vi "Guarda_Datos.vi"(0 "Texto (I)":string, 1 "Ruta":path, 2 "Operación":T1(ring), 3 "Acceso":enum16{"read/write", "read-only", "write-only"}(ring), 4 "Error (I)":errorcluster) -> (5 "Texto (O)":string, 6 "Error (O)":errorcluster)   [LabVIEW 2020]
doc: "Selecciona la operación que se quiere ejecutar sobre el archivo especificado en la ruta y el tipo de acceso que se desea tener a él, para escribir el texto entregado y/o leer el texto en el mismo. La operación de lectura y escritura ocurre en ese orden: lectura y luego escritura.\n\nTexto (I): Texto que será escrito al final del archivo.\n\nRuta: Ruta del archivo (el archivo mismo y su extensión es parte de la ruta).\n\nOperación: 0 - Abrir; 1 - Reemplazar; 2 - Crear; 3 - Abrir o crear; 4 - Reemplazar o crear; 5 - Reemplazar o creear con confirmación.\n\nAcceso: 0 - Leer y Escribir; 1 - Leer; 2 - Escribir.\n\nError (I): Ingreso de errores previos.\n\nTexto (O): Texto contenido en el archivo antes de escribirle el nuevo texto en Texto (I). Devuelve un string explicando un error en caso de que el Acceso no permita la opción de Leer.\n\nError (O): Salida de errores previos más los de esta VI."
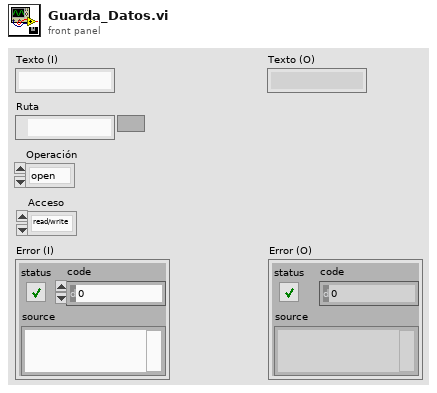
[diagram p1: front panel]
types:
  T1 = enum16{"open", "replace", "create", "open or create", "replace or create", "replace or create with confirmation"}
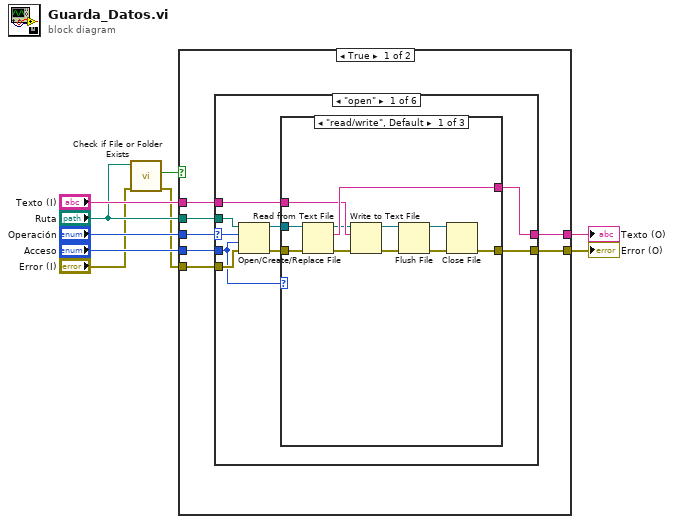
[diagram p0: block diagram]
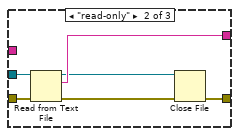
[diagram p2: hidden frame]
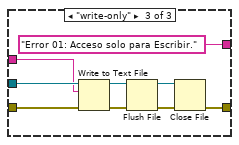
[diagram p3: hidden frame]
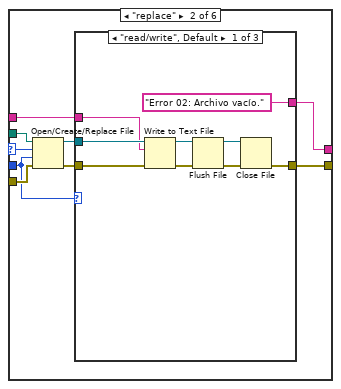
[diagram p4: hidden frame]
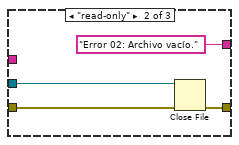
[diagram p5: hidden frame]
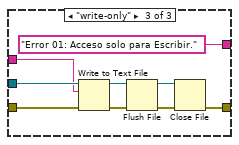
[diagram p6: hidden frame]
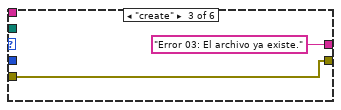
[diagram p7: hidden frame]
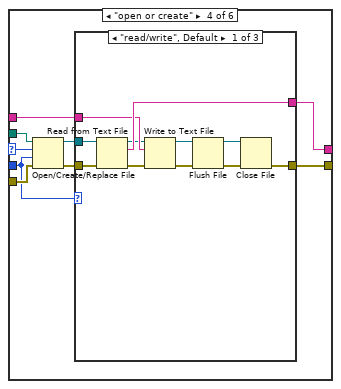
[diagram p8: hidden frame]
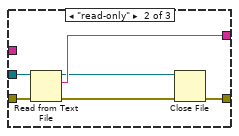
[diagram p9: hidden frame]
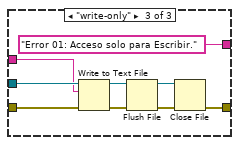
[diagram p10: hidden frame]
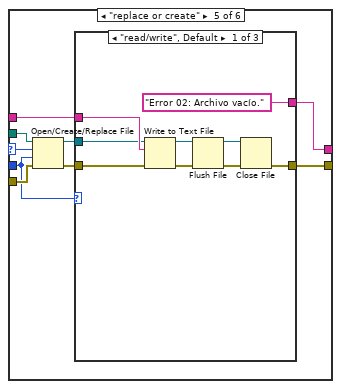
[diagram p11: hidden frame]
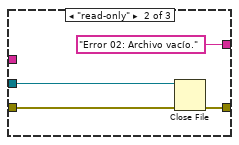
[diagram p12: hidden frame]
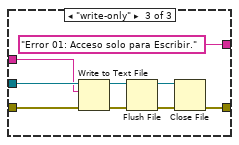
[diagram p13: hidden frame]
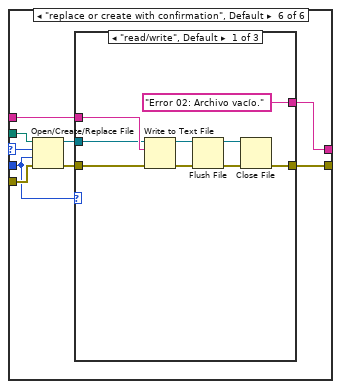
[diagram p14: hidden frame]
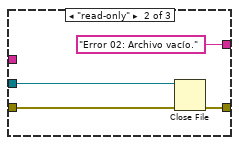
[diagram p15: hidden frame]
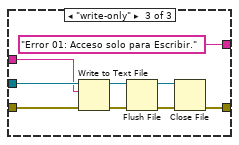
[diagram p16: hidden frame]
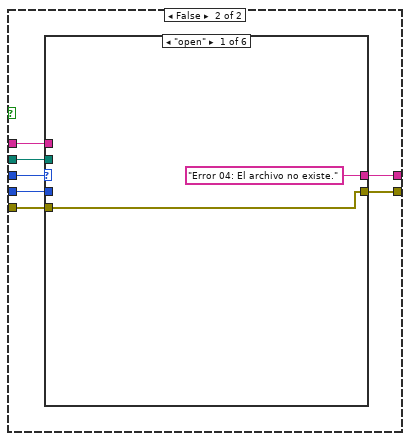
[diagram p17: hidden frame]
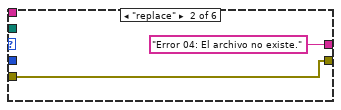
[diagram p18: hidden frame]
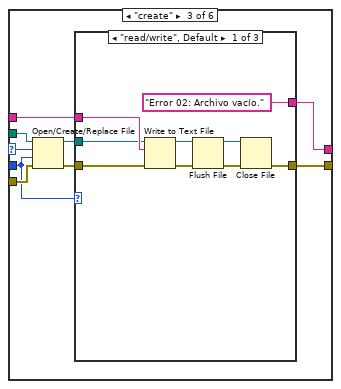
[diagram p19: hidden frame]
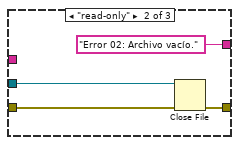
[diagram p20: hidden frame]
diagram:
  n1 = call <vilib>:"Check if File or Folder Exists.vi"("error in (no error)"="Error (I)", "path"="Ruta") -> ("error out"=w1:errorcluster, "file or folder exists?"=w3:bool)  [unwired: 7 in, 1 out]
  n2 = case shown="True" w3 {
    tunnel: "Operación" -> [w16 w188]
    tunnel: "Ruta" -> [w15 w187]
    tunnel: "Acceso" -> [w14 w186]
    tunnel: w1 -> [w13 w185]
    tunnel: "Texto (I)" -> [w12 w184]
    tunnel: [w11 w183] -> w6
    tunnel: [w10 w182] -> w5
    frame True {
      n3 = case shown="\"open\"" w16 {
        selector: w16 -> [w25 w60 _ w93 w128 w159]
        tunnel: w15 -> [w24 w59 _ w92 w127 w158]
        tunnel: w14 -> [w22 w57 _ w90 w125 w156]
        tunnel: w13 -> [w23 w58 w84 w91 w126 w157]
        tunnel: w12 -> [w19 w54 _ w87 w122 w153]
        tunnel: [w18 w53 w84 w86 w121 w152] -> w11
        tunnel: [w17 w52 "Error 03: El archivo ya existe." ("Texto (I)") w85 w120 w151] -> w10
        frame "open" {
          n4 = Open/Create/Replace File(file path (use dialog)=w24, error in=w23, operation (0:open)=w25, access (0:read/write)=w22) -> (refnum out=w21:refnum<file>, error out=w20:errorcluster)  [unwired: 2 in, 1 out]
          n5 = case shown="\"read/write\", Default" w22 {
            tunnel: w21 -> [w36 w42 w46]
            tunnel: w20 -> [w35 w41 w45]
            tunnel: [w34 w40 "Error 01: Acceso solo para Escribir."] -> w17
            tunnel: w19 -> [w33 _ w44]
            tunnel: [w26 w39 w47] -> w18
            frame "read/write", Default {
              n6 = Read from Text File(file (use dialog)=w36, error in=w35) -> (refnum out=w32:refnum<file>, text=w34:string, error out=w31:errorcluster)  [unwired: 2 in, 1 out]
              n7 = Write to Text File(file (use dialog)=w32, text=w33, error in=w31) -> (refnum out=w30:refnum<file>, error out=w29:errorcluster)  [unwired: 1 in, 1 out]
              n8 = Flush File(refnum=w30, error in=w29) -> (refnum out=w28:refnum<file>, error out=w27:errorcluster)
              n9 = Close File(refnum=w28, error in=w27) -> (error out=w26:errorcluster)  [unwired: 1 out]
            }
            frame "read-only" {
              n10 = Read from Text File(file (use dialog)=w42, error in=w41) -> (refnum out=w37:refnum<file>, text=w40:string, error out=w38:errorcluster)  [unwired: 2 in, 1 out]
              n11 = Close File(refnum=w37, error in=w38) -> (error out=w39:errorcluster)  [unwired: 1 out]
            }
            frame "write-only" {
              n12 = Write to Text File(file (use dialog)=w46, text=w44, error in=w45) -> (refnum out=w51:refnum<file>, error out=w50:errorcluster)  [unwired: 1 in, 1 out]
              n13 = Flush File(refnum=w51, error in=w50) -> (refnum out=w49:refnum<file>, error out=w48:errorcluster)
              n14 = Close File(refnum=w49, error in=w48) -> (error out=w47:errorcluster)  [unwired: 1 out]
            }
          }
        }
        frame "replace" {
          n15 = Open/Create/Replace File(file path (use dialog)=w59, error in=w58, operation (0:open)=w60, access (0:read/write)=w57) -> (refnum out=w56:refnum<file>, error out=w55:errorcluster)  [unwired: 2 in, 1 out]
          n16 = case shown="\"read/write\", Default" w57 {
            tunnel: w56 -> [w65 w71 w77]
            tunnel: w55 -> [w64 w72 w76]
            tunnel: ["Error 02: Archivo vacío." ("Texto (I)") "Error 02: Archivo vacío." ("Texto (I)") "Error 01: Acceso solo para Escribir." ("Texto (I)")] -> w52
            tunnel: w54 -> [w62 _ w75]
            tunnel: [w63 w70 w78] -> w53
            frame "read/write", Default {
              n17 = Write to Text File(file (use dialog)=w65, text=w62, error in=w64) -> (refnum out=w69:refnum<file>, error out=w68:errorcluster)  [unwired: 1 in, 1 out]
              n18 = Flush File(refnum=w69, error in=w68) -> (refnum out=w67:refnum<file>, error out=w66:errorcluster)
              n19 = Close File(refnum=w67, error in=w66) -> (error out=w63:errorcluster)  [unwired: 1 out]
            }
            frame "read-only" {
              n20 = Close File(refnum=w71, error in=w72) -> (error out=w70:errorcluster)  [unwired: 1 out]
            }
            frame "write-only" {
              n21 = Write to Text File(file (use dialog)=w77, text=w75, error in=w76) -> (refnum out=w82:refnum<file>, error out=w81:errorcluster)  [unwired: 1 in, 1 out]
              n22 = Flush File(refnum=w82, error in=w81) -> (refnum out=w80:refnum<file>, error out=w79:errorcluster)
              n23 = Close File(refnum=w80, error in=w79) -> (error out=w78:errorcluster)  [unwired: 1 out]
            }
          }
        }
        frame "create" {
        }
        frame "open or create" {
          n24 = Open/Create/Replace File(file path (use dialog)=w92, error in=w91, operation (0:open)=w93, access (0:read/write)=w90) -> (refnum out=w89:refnum<file>, error out=w88:errorcluster)  [unwired: 2 in, 1 out]
          n25 = case shown="\"read/write\", Default" w90 {
            tunnel: w89 -> [w104 w110 w114]
            tunnel: w88 -> [w103 w109 w113]
            tunnel: [w102 w108 "Error 01: Acceso solo para Escribir."] -> w85
            tunnel: w87 -> [w101 _ w112]
            tunnel: [w94 w107 w115] -> w86
            frame "read/write", Default {
              n26 = Read from Text File(file (use dialog)=w104, error in=w103) -> (refnum out=w100:refnum<file>, text=w102:string, error out=w99:errorcluster)  [unwired: 2 in, 1 out]
              n27 = Write to Text File(file (use dialog)=w100, text=w101, error in=w99) -> (refnum out=w98:refnum<file>, error out=w97:errorcluster)  [unwired: 1 in, 1 out]
              n28 = Flush File(refnum=w98, error in=w97) -> (refnum out=w96:refnum<file>, error out=w95:errorcluster)
              n29 = Close File(refnum=w96, error in=w95) -> (error out=w94:errorcluster)  [unwired: 1 out]
            }
            frame "read-only" {
              n30 = Read from Text File(file (use dialog)=w110, error in=w109) -> (refnum out=w105:refnum<file>, text=w108:string, error out=w106:errorcluster)  [unwired: 2 in, 1 out]
              n31 = Close File(refnum=w105, error in=w106) -> (error out=w107:errorcluster)  [unwired: 1 out]
            }
            frame "write-only" {
              n32 = Write to Text File(file (use dialog)=w114, text=w112, error in=w113) -> (refnum out=w119:refnum<file>, error out=w118:errorcluster)  [unwired: 1 in, 1 out]
              n33 = Flush File(refnum=w119, error in=w118) -> (refnum out=w117:refnum<file>, error out=w116:errorcluster)
              n34 = Close File(refnum=w117, error in=w116) -> (error out=w115:errorcluster)  [unwired: 1 out]
            }
          }
        }
        frame "replace or create" {
          n35 = Open/Create/Replace File(file path (use dialog)=w127, error in=w126, operation (0:open)=w128, access (0:read/write)=w125) -> (refnum out=w124:refnum<file>, error out=w123:errorcluster)  [unwired: 2 in, 1 out]
          n36 = case shown="\"read/write\", Default" w125 {
            tunnel: w124 -> [w131 w138 w145]
            tunnel: w123 -> [w130 w140 w144]
            tunnel: ["Error 02: Archivo vacío." ("Texto (I)") "Error 02: Archivo vacío." ("Texto (I)") "Error 01: Acceso solo para Escribir." ("Texto (I)")] -> w120
            tunnel: w122 -> [w132 _ w143]
            tunnel: [w133 w139 w146] -> w121
            frame "read/write", Default {
              n37 = Write to Text File(file (use dialog)=w131, text=w132, error in=w130) -> (refnum out=w137:refnum<file>, error out=w136:errorcluster)  [unwired: 1 in, 1 out]
              n38 = Flush File(refnum=w137, error in=w136) -> (refnum out=w135:refnum<file>, error out=w134:errorcluster)
              n39 = Close File(refnum=w135, error in=w134) -> (error out=w133:errorcluster)  [unwired: 1 out]
            }
            frame "read-only" {
              n40 = Close File(refnum=w138, error in=w140) -> (error out=w139:errorcluster)  [unwired: 1 out]
            }
            frame "write-only" {
              n41 = Write to Text File(file (use dialog)=w145, text=w143, error in=w144) -> (refnum out=w150:refnum<file>, error out=w149:errorcluster)  [unwired: 1 in, 1 out]
              n42 = Flush File(refnum=w150, error in=w149) -> (refnum out=w148:refnum<file>, error out=w147:errorcluster)
              n43 = Close File(refnum=w148, error in=w147) -> (error out=w146:errorcluster)  [unwired: 1 out]
            }
          }
        }
        frame "replace or create with confirmation", Default {
          n44 = Open/Create/Replace File(file path (use dialog)=w158, error in=w157, operation (0:open)=w159, access (0:read/write)=w156) -> (refnum out=w155:refnum<file>, error out=w154:errorcluster)  [unwired: 2 in, 1 out]
          n45 = case shown="\"read/write\", Default" w156 {
            tunnel: w155 -> [w162 w169 w176]
            tunnel: w154 -> [w161 w170 w175]
            tunnel: ["Error 02: Archivo vacío." ("Texto (I)") "Error 02: Archivo vacío." ("Texto (I)") "Error 01: Acceso solo para Escribir." ("Texto (I)")] -> w151
            tunnel: w153 -> [w163 _ w174]
            tunnel: [w164 w171 w177] -> w152
            frame "read/write", Default {
              n46 = Write to Text File(file (use dialog)=w162, text=w163, error in=w161) -> (refnum out=w168:refnum<file>, error out=w167:errorcluster)  [unwired: 1 in, 1 out]
              n47 = Flush File(refnum=w168, error in=w167) -> (refnum out=w166:refnum<file>, error out=w165:errorcluster)
              n48 = Close File(refnum=w166, error in=w165) -> (error out=w164:errorcluster)  [unwired: 1 out]
            }
            frame "read-only" {
              n49 = Close File(refnum=w169, error in=w170) -> (error out=w171:errorcluster)  [unwired: 1 out]
            }
            frame "write-only" {
              n50 = Write to Text File(file (use dialog)=w176, text=w174, error in=w175) -> (refnum out=w181:refnum<file>, error out=w180:errorcluster)  [unwired: 1 in, 1 out]
              n51 = Flush File(refnum=w181, error in=w180) -> (refnum out=w179:refnum<file>, error out=w178:errorcluster)
              n52 = Close File(refnum=w179, error in=w178) -> (error out=w177:errorcluster)  [unwired: 1 out]
            }
          }
        }
      }
    }
    frame False {
      n53 = case shown="\"open\"" w188 {
        selector: w188 -> [_ _ w200 w232 w263 w294]
        tunnel: w187 -> [_ _ w198 w231 w262 w293]
        tunnel: w186 -> [_ _ w194 w229 w260 w291]
        tunnel: w185 -> [w190 w192 w197 w230 w261 w292]
        tunnel: w184 -> [_ _ w199 w226 w257 w288]
        tunnel: [w190 w192 w201 w225 w256 w287] -> w183
        tunnel: ["Error 04: El archivo no existe." ("Texto (I)") "Error 04: El archivo no existe." ("Texto (I)") w193 w224 w255 w286] -> w182
        frame "open" {
        }
        frame "replace" {
        }
        frame "create" {
          n54 = Open/Create/Replace File(file path (use dialog)=w198, error in=w197, operation (0:open)=w200, access (0:read/write)=w194) -> (refnum out=w196:refnum<file>, error out=w195:errorcluster)  [unwired: 2 in, 1 out]
          n55 = case shown="\"read/write\", Default" w194 {
            tunnel: w196 -> [w203 w212 w218]
            tunnel: w195 -> [w202 w211 w217]
            tunnel: ["Error 02: Archivo vacío." "Error 02: Archivo vacío." "Error 01: Acceso solo para Escribir."] -> w193
            tunnel: w199 -> [w210 _ w216]
            tunnel: [w205 w214 w219] -> w201
            frame "read/write", Default {
              n56 = Write to Text File(file (use dialog)=w203, text=w210, error in=w202) -> (refnum out=w209:refnum<file>, error out=w208:errorcluster)  [unwired: 1 in, 1 out]
              n57 = Flush File(refnum=w209, error in=w208) -> (refnum out=w207:refnum<file>, error out=w206:errorcluster)
              n58 = Close File(refnum=w207, error in=w206) -> (error out=w205:errorcluster)  [unwired: 1 out]
            }
            frame "read-only" {
              n59 = Close File(refnum=w212, error in=w211) -> (error out=w214:errorcluster)  [unwired: 1 out]
            }
            frame "write-only" {
              n60 = Write to Text File(file (use dialog)=w218, text=w216, error in=w217) -> (refnum out=w223:refnum<file>, error out=w222:errorcluster)  [unwired: 1 in, 1 out]
              n61 = Flush File(refnum=w223, error in=w222) -> (refnum out=w221:refnum<file>, error out=w220:errorcluster)
              n62 = Close File(refnum=w221, error in=w220) -> (error out=w219:errorcluster)  [unwired: 1 out]
            }
          }
        }
        frame "open or create" {
          n63 = Open/Create/Replace File(file path (use dialog)=w231, error in=w230, operation (0:open)=w232, access (0:read/write)=w229) -> (refnum out=w228:refnum<file>, error out=w227:errorcluster)  [unwired: 2 in, 1 out]
          n64 = case shown="\"read/write\", Default" w229 {
            tunnel: w228 -> [w235 w244 w249]
            tunnel: w227 -> [w234 w243 w248]
            tunnel: ["Error 02: Archivo vacío." "Error 02: Archivo vacío." "Error 01: Acceso solo para Escribir."] -> w224
            tunnel: w226 -> [w241 _ w247]
            tunnel: [w236 w245 w250] -> w225
            frame "read/write", Default {
              n65 = Write to Text File(file (use dialog)=w235, text=w241, error in=w234) -> (refnum out=w240:refnum<file>, error out=w239:errorcluster)  [unwired: 1 in, 1 out]
              n66 = Flush File(refnum=w240, error in=w239) -> (refnum out=w238:refnum<file>, error out=w237:errorcluster)
              n67 = Close File(refnum=w238, error in=w237) -> (error out=w236:errorcluster)  [unwired: 1 out]
            }
            frame "read-only" {
              n68 = Close File(refnum=w244, error in=w243) -> (error out=w245:errorcluster)  [unwired: 1 out]
            }
            frame "write-only" {
              n69 = Write to Text File(file (use dialog)=w249, text=w247, error in=w248) -> (refnum out=w254:refnum<file>, error out=w253:errorcluster)  [unwired: 1 in, 1 out]
              n70 = Flush File(refnum=w254, error in=w253) -> (refnum out=w252:refnum<file>, error out=w251:errorcluster)
              n71 = Close File(refnum=w252, error in=w251) -> (error out=w250:errorcluster)  [unwired: 1 out]
            }
          }
        }
        frame "replace or create" {
          n72 = Open/Create/Replace File(file path (use dialog)=w262, error in=w261, operation (0:open)=w263, access (0:read/write)=w260) -> (refnum out=w259:refnum<file>, error out=w258:errorcluster)  [unwired: 2 in, 1 out]
          n73 = case shown="\"read/write\", Default" w260 {
            tunnel: w259 -> [w266 w273 w280]
            tunnel: w258 -> [w265 w274 w279]
            tunnel: ["Error 02: Archivo vacío." ("Texto (I)") "Error 02: Archivo vacío." ("Texto (I)") "Error 01: Acceso solo para Escribir." ("Texto (I)")] -> w255
            tunnel: w257 -> [w267 _ w278]
            tunnel: [w268 w275 w281] -> w256
            frame "read/write", Default {
              n74 = Write to Text File(file (use dialog)=w266, text=w267, error in=w265) -> (refnum out=w272:refnum<file>, error out=w271:errorcluster)  [unwired: 1 in, 1 out]
              n75 = Flush File(refnum=w272, error in=w271) -> (refnum out=w270:refnum<file>, error out=w269:errorcluster)
              n76 = Close File(refnum=w270, error in=w269) -> (error out=w268:errorcluster)  [unwired: 1 out]
            }
            frame "read-only" {
              n77 = Close File(refnum=w273, error in=w274) -> (error out=w275:errorcluster)  [unwired: 1 out]
            }
            frame "write-only" {
              n78 = Write to Text File(file (use dialog)=w280, text=w278, error in=w279) -> (refnum out=w285:refnum<file>, error out=w284:errorcluster)  [unwired: 1 in, 1 out]
              n79 = Flush File(refnum=w285, error in=w284) -> (refnum out=w283:refnum<file>, error out=w282:errorcluster)
              n80 = Close File(refnum=w283, error in=w282) -> (error out=w281:errorcluster)  [unwired: 1 out]
            }
          }
        }
        frame "replace or create with confirmation", Default {
          n81 = Open/Create/Replace File(file path (use dialog)=w293, error in=w292, operation (0:open)=w294, access (0:read/write)=w291) -> (refnum out=w290:refnum<file>, error out=w289:errorcluster)  [unwired: 2 in, 1 out]
          n82 = case shown="\"read/write\", Default" w291 {
            tunnel: w290 -> [w297 w304 w311]
            tunnel: w289 -> [w296 w306 w310]
            tunnel: ["Error 02: Archivo vacío." ("Texto (I)") "Error 02: Archivo vacío." ("Texto (I)") "Error 01: Acceso solo para Escribir." ("Texto (I)")] -> w286
            tunnel: w288 -> [w298 _ w309]
            tunnel: [w299 w305 w312] -> w287
            frame "read/write", Default {
              n83 = Write to Text File(file (use dialog)=w297, text=w298, error in=w296) -> (refnum out=w303:refnum<file>, error out=w302:errorcluster)  [unwired: 1 in, 1 out]
              n84 = Flush File(refnum=w303, error in=w302) -> (refnum out=w301:refnum<file>, error out=w300:errorcluster)
              n85 = Close File(refnum=w301, error in=w300) -> (error out=w299:errorcluster)  [unwired: 1 out]
            }
            frame "read-only" {
              n86 = Close File(refnum=w304, error in=w306) -> (error out=w305:errorcluster)  [unwired: 1 out]
            }
            frame "write-only" {
              n87 = Write to Text File(file (use dialog)=w311, text=w309, error in=w310) -> (refnum out=w316:refnum<file>, error out=w315:errorcluster)  [unwired: 1 in, 1 out]
              n88 = Flush File(refnum=w316, error in=w315) -> (refnum out=w314:refnum<file>, error out=w313:errorcluster)
              n89 = Close File(refnum=w314, error in=w313) -> (error out=w312:errorcluster)  [unwired: 1 out]
            }
          }
        }
      }
    }
  }
  "Error (O)" <- w6
  "Texto (O)" <- w5
